vi "ma_align N waveforms (common interval with remainder).vi"(0 "waveforms in":waveform(dbl)[](array[waveform]), 11 "error in":errorcluster) -> (4 "intersecting waveforms out":waveform(dbl)[](array[waveform]), 6 "remainder waveforms out":waveform(dbl)[](array[waveform]), 15 "error out":errorcluster)   [LabVIEW 2020, in "NI_MAPro.lvlib"]
uses:
  NI_MAPro.lvlib
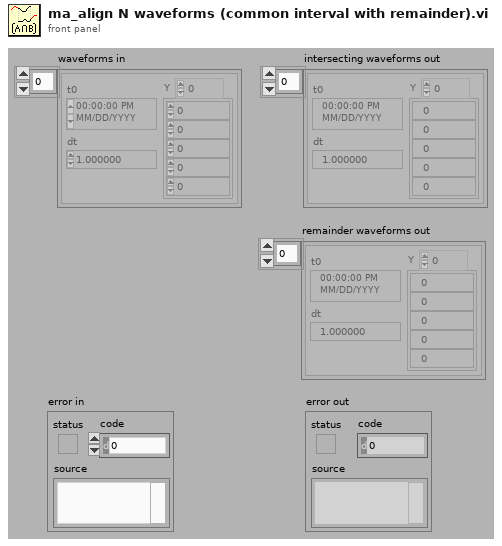
[diagram p1: front panel]
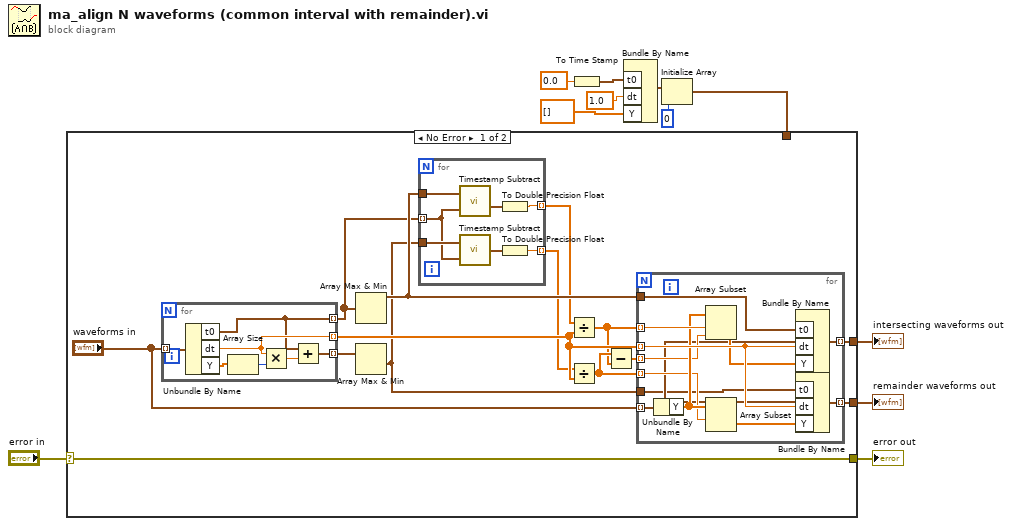
[diagram p0: block diagram]
diagram:
  n1 = To Time Stamp(1:0.0 ("t0")) -> (0:w1:timestamp)
  n2 = Bundle By Name("t0"=w1, "dt"=1.0, "Y"=dbl[] []) -> (w7:waveform(dbl))  [unwired: 1 in]
  n3 = Initialize Array(w7, 0 ("dimension size")) -> (w3:waveform(dbl)[])
  n4 = case shown="No Error" "error in" {
    selector: "error in" -> [w25 w53]
    tunnel: [w25 w53] -> w11
    tunnel: [w24 w52] -> w9
    tunnel: w3 -> [_ w52]
    tunnel: [w22 w52] -> w2
    frame No Error {
      n5 = for {
        tunnel: "waveforms in" -> [w39] mode=indexing
        tunnel: [w37] -> w19 mode=indexing
        tunnel: [w33] -> w17 mode=indexing
        tunnel: [w35] -> w21 mode=indexing
        n6 = Unbundle By Name(w39) -> ("t0"=w33:timestamp, "dt"=w35:dbl, "Y"=w36:dbl[])
        n7 = Array Size(array=w36) -> (size(s)=w34:i32)
        n8 = Multiply(x=w35, y=w34) -> (x*y=w38:dbl)
        n9 = Add(x=w33, y=w38) -> (x+y=w37:timestamp)
      }
      n10 = Array Max & Min(array=w17) -> (max value=w20:timestamp)  [unwired: 3 out]
      n11 = Array Max & Min(array=w19) -> (min value=w18:timestamp)  [unwired: 3 out]
      n12 = for {
        tunnel: w20 -> [w30]
        tunnel: w18 -> [w29]
        tunnel: w17 -> [w28] mode=indexing
        tunnel: [w27] -> w13 mode=indexing
        tunnel: [w26] -> w12 mode=indexing
        n13 = call "Timestamp Subtract.vi"("y"=w28, "x"=w30) -> ("x - y"=w31:timestamp)
        n14 = call "Timestamp Subtract.vi"("y"=w28, "x"=w29) -> ("x - y"=w32:timestamp)
        n15 = To Double Precision Float(number=w31) -> (double precision float=w27:dbl)
        n16 = To Double Precision Float(number=w32) -> (double precision float=w26:dbl)
      }
      n17 = Divide(x=w13, y=w21) -> (x/y=w15:dbl[])
      n18 = Divide(x=w12, y=w21) -> (x/y=w16:dbl[])
      n19 = Subtract(x=w16, y=w15) -> (x-y=w14:dbl[])
      n20 = for {
        tunnel: "waveforms in" -> [w42] mode=indexing
        tunnel: w15 -> [w48] mode=indexing
        tunnel: w16 -> [w46] mode=indexing
        tunnel: w21 -> [w50] mode=indexing
        tunnel: w20 -> [w41]
        tunnel: [w51] -> w24 mode=indexing
        tunnel: w18 -> [w40]
        tunnel: [w49] -> w22 mode=indexing
        tunnel: w14 -> [w44] mode=indexing
        n21 = Unbundle By Name(w42) -> ("Y"=w47:dbl[])
        n22 = Array Subset(array=w47, index=w48, length=w44) -> (w43:dbl[])
        n23 = Array Subset(array=w47, index=w46) -> (w45:dbl[])  [unwired: 1 in]
        n24 = Bundle By Name(cluster=w42, "t0"=w41, "dt"=w50, "Y"=w43) -> (w51:waveform(dbl))
        n25 = Bundle By Name(cluster=w42, "t0"=w40, "dt"=w50, "Y"=w45) -> (w49:waveform(dbl))
      }
    }
    frame Error {
    }
  }
  "error out" <- w11
  "intersecting waveforms out" <- w9
  "remainder waveforms out" <- w2
